vi "Invert In-Place (Greyscale Bitwise).vi"(8 "error in (no error)":errorcluster, 11 "Greyscale Image to Invert in Place in":T1) -> (0 "error out":errorcluster, 3 "Greyscale Image":T1)   [LabVIEW 2020, in "image.lvlib"]
doc: "Invert the Pixels in the Greyscale Image in-place.\n\nThis function is useful when inverting a Greyscale Image which represents a mask."
uses:
  image.lvlib
  821d400d-177f-4d99-a785-a8086a4d8ddd.vi
  Greyscale Image.ctl
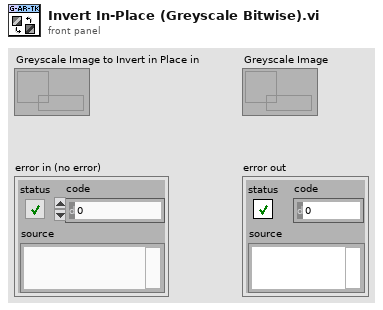
[diagram p1: front panel]
types:
  T1 = typedef "image.lvlib/Greyscale Image.ctl" = refnum<data-value>
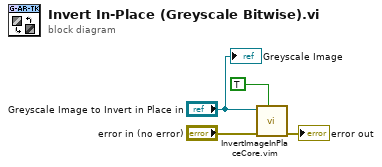
[diagram p0: block diagram]
diagram:
  n1 = call "InvertImageInPlaceCore.vim"("Use Bitwise"=TRUE, "error in (no error)"="error in (no error)", "Image In"="Greyscale Image to Invert in Place in") -> ("error out"=→"error out":errorcluster)  [unwired: 8 in]
  "Greyscale Image" <- "Greyscale Image to Invert in Place in"
